vi "sv_Subtract U32 Integers.vi"(9 "y (U32)":u32, 10 "x (U32)":u32) -> (2 "x-y (U32)":u32)   [LabVIEW 2017]
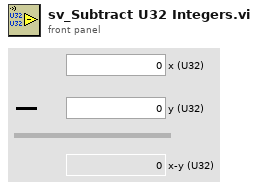
[diagram p1: front panel]
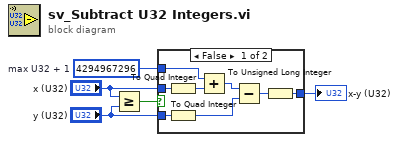
[diagram p0: block diagram]
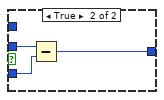
[diagram p2: hidden frame]
diagram:
  w1 = i64 4294967296  # max U32 + 1
  n1 = Greater Or Equal?(x="x (U32)", y="y (U32)") -> (x >= y?=w2:bool)
  n2 = case shown="False" w2 {
    tunnel: [w8 w16] -> w5
    tunnel: "x (U32)" -> [w13 w15]
    tunnel: "y (U32)" -> [w9 w14]
    tunnel: w1 -> [w10 _]
    frame False {
      n3 = To Quad Integer(1:w13) -> (0:w12:i64)
      n4 = To Quad Integer(1:w9) -> (0:w7:i64)
      n5 = Add(x=w10, y=w12) -> (x+y=w11:i64)
      n6 = Subtract(x=w11, y=w7) -> (x-y=w6:i64)
      n7 = To Unsigned Long Integer(number=w6) -> (unsigned 32bit integer=w8:u32)
    }
    frame True {
      n8 = Subtract(x=w15, y=w14) -> (x-y=w16:u32)
    }
  }
  "x-y (U32)" <- w5
